vi "Read Data Type.vi"(8 "error in (no error)":errorcluster, 11 "Update Tag in":refnum<class "Update Tag Config.lvclass">) -> (0 "error out":errorcluster, 2 "data type":T1, 3 "Update Tag out":refnum<class "Update Tag Config.lvclass">)   [LabVIEW 2015]
uses:
  Update Tag Config.lvclass
  <vilib>/NI/Tag Bus/tag/Data Type.ctl
  <vilib>/NI/Tag Bus/tag/tag descriptor.lvclass
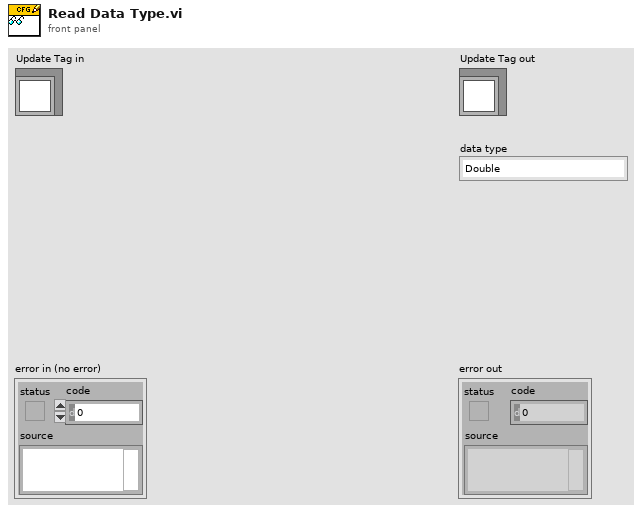
[diagram p1: front panel]
types:
  T1 = typedef "tag bus.lvlib/tag descriptor.lvclass/Data Type.ctl" = enum16{"Double", "Single", "I64", "I32", "I16", "I8", "U64", "U32", "U16", "U8", "Boolean", "String", "Array of Double", "Array of Single", "Array of I64", "Array of I32", "Array of I16", "Array of I8", "Array of U64", "Array of U32", "Array of U16", "Array of U8", "Array of Boolean", "Array of String"}
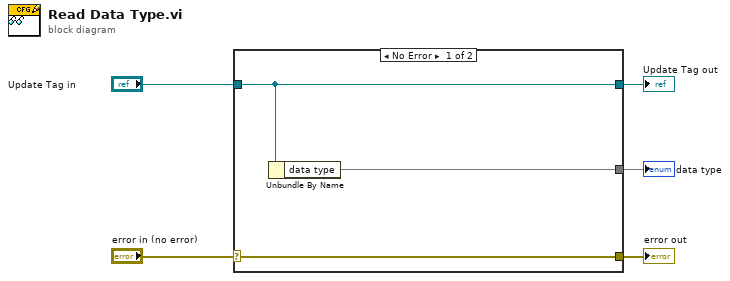
[diagram p0: block diagram]
diagram:
  n1 = case shown="No Error" "error in (no error)" {
    selector: "error in (no error)" -> [w8 w9]
    tunnel: [w8 w9] -> w4
    tunnel: [w7 w10] -> w2
    tunnel: "Update Tag in" -> [w7 w10]
    tunnel: [w6 _] -> w1
    frame No Error {
      n2 = Unbundle By Name(w7) -> ("data type"=w6)
    }
    frame Error {
    }
  }
  "error out" <- w4
  "Update Tag out" <- w2
  "data type" <- w1
